vi "SetMCP.vi"(0 "Strings in":string[](array[string])=["C:\\CuspControl\\GPIB and Network\\Cusp\\MCPvolts.txt", "6723"], 1 "Dubs in":dbl[](array[numeric])=[0.0, 0.0, 0.0]) -> ()   [LabVIEW 2018]
panel:
  in  "Tab Control":enum32{"Variables", "Setup"}(tab)
  in  "Gain (Vout/Vcontrol)":dbl[](array[numeric])=[15.0, 208.0, 511.0]
  in  "mcpF, mcpB, phos (end)":dbl[](array[numeric])=[0.0, 0.0, 0.0] format="%0.2f"
  in  "mcpF, mcpB, phos (start)":dbl[](array[numeric])=[0.0, 0.0, 0.0] format="%0.2f"
  in  "upper limit":dbl[](array[numeric])=[100.0, 900.0, 3200.0]
  in  "lower limit":dbl[](array[numeric])=[-100.0, 0.0, 0.0]
  in  "MCPvolts":path=path "C:/CuspControl/GPIB and Network/Cusp/MCPvolts.txt"
  in  "ao lines":string[](array[string])=["ao5", "ao6", "ao7"]
  in  "subvi":bool=TRUE
  in  "gain file":path=path "C:/CuspControl/Cusp/Configuration/MCPgain.txt"
  # "DO NOT CHANGE GAIN"
  # "ao5\nao6\nao7"
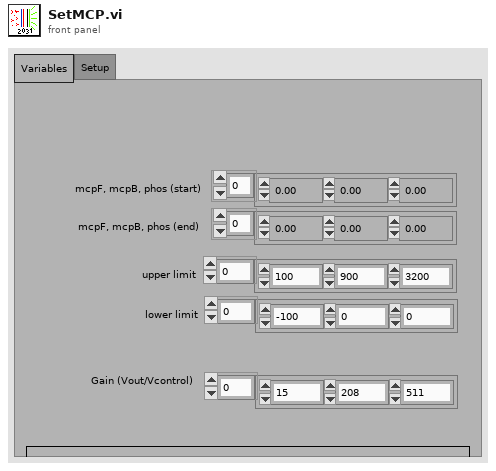
[diagram p1: front panel]
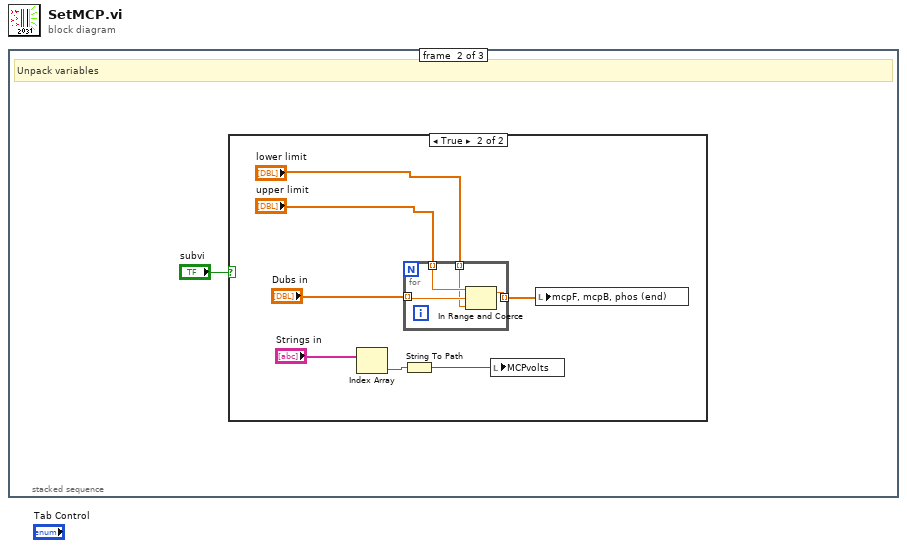
[diagram p0: block diagram]
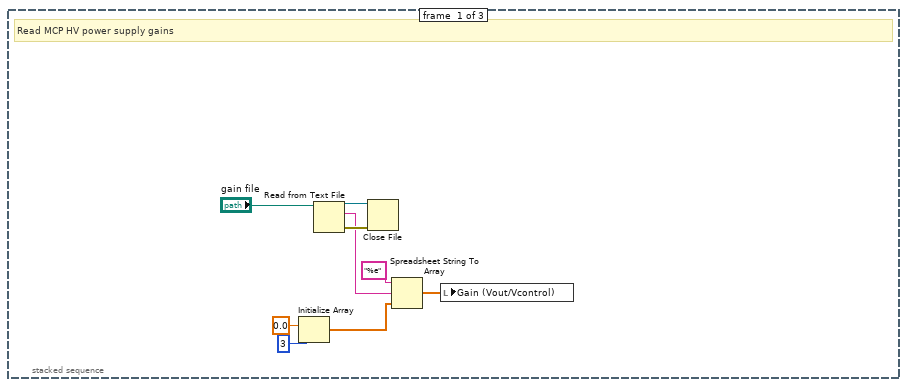
[diagram p2: hidden frame]
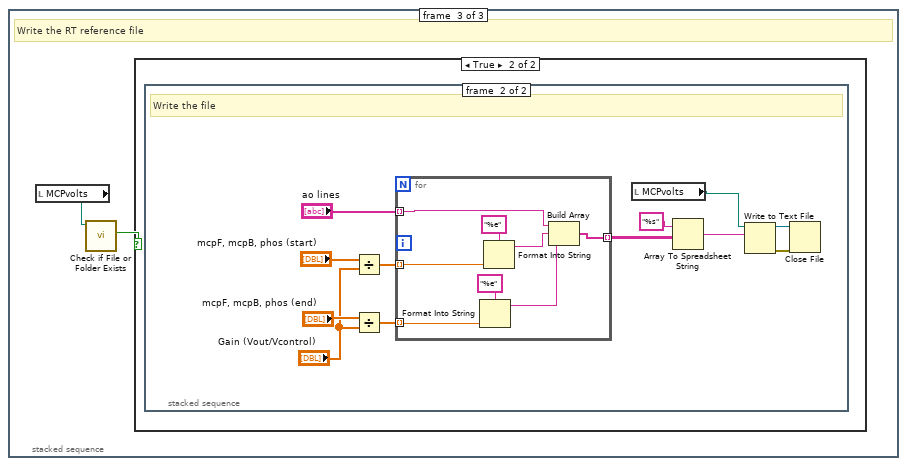
[diagram p4: hidden frame]
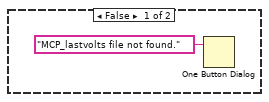
[diagram p5: hidden frame]
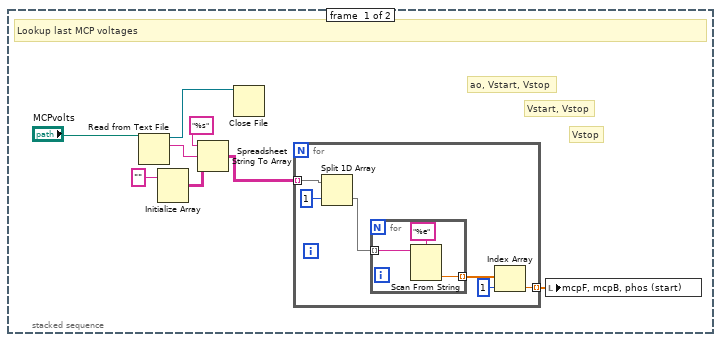
[diagram p6: hidden frame]
diagram:
  n1 = stacked-sequence {
    frame #0 {
      # "Read MCP HV power supply gains"
      n2 = Initialize Array(0.0 ("element"), 3 ("dimension size")) -> (w3:dbl[])
      n3 = Read from Text File(file (use dialog)="gain file") -> (refnum out=w8:refnum<file>, text=w6:string, error out=w7:errorcluster)  [unwired: 3 in, 1 out]
      n4 = Close File(refnum=w8, error in=w7) -> ()  [unwired: 2 out]
      n5 = Spreadsheet String To Array(format string="%e", spreadsheet string=w6, array type (2D Dbl)=w3) -> (array=w1:dbl[])  [unwired: 1 in]
      n6 = local write "Gain (Vout/Vcontrol)"(w1) -> ()
    }
    frame #1 {
      # "Unpack variables"
      n7 = case shown="True" "subvi" {
        frame False {
        }
        frame True {
          n8 = Index Array(array="Strings in") -> (element=w16:string)  [unwired: 1 in]
          n9 = for {
            tunnel: "Dubs in" -> [w21] mode=indexing
            tunnel: [w20] -> w13 mode=indexing
            tunnel: "upper limit" -> [w19] mode=indexing
            tunnel: "lower limit" -> [w18] mode=indexing
            n10 = In Range and Coerce(upper limit=w19, x=w21, lower limit=w18) -> (coerced(x)=w20:dbl)  [unwired: 1 out]
          }
          n11 = String To Path(string=w16) -> (path=w15:path)
          n12 = local write "MCPvolts"(w15) -> ()
          n13 = local write "mcpF, mcpB, phos (end)"(w13) -> ()
        }
      }
    }
    frame #2 {
      # "Write the RT reference file"
      n14 = local read "MCPvolts"() -> (w23:path)
      n15 = call <vilib>:"Check if File or Folder Exists.vi"("path"=w23) -> ("file or folder exists?"=w22:bool)  [unwired: 8 in, 2 out]
      n16 = case shown="True" w22 {
        frame False {
          n17 = One Button Dialog(message="MCP_lastvolts file not found.") -> ()  [unwired: 1 in, 1 out]
        }
        frame True {
          n18 = stacked-sequence {
            frame #0 {
              # "Vstop"
              # "Vstart, Vstop"
              # "ao, Vstart, Vstop"
              # "Lookup last MCP voltages"
              n19 = Read from Text File(file (use dialog)="MCPvolts") -> (refnum out=w27:refnum<file>, text=w28:string)  [unwired: 3 in, 2 out]
              n20 = Initialize Array("") -> (w30:string[][])  [unwired: 2 in]
              n21 = Spreadsheet String To Array(format string="%s", spreadsheet string=w28, array type (2D Dbl)=w30) -> (array=w32:string[][])  [unwired: 1 in]
              n22 = Close File(refnum=w27) -> ()  [unwired: 1 in, 2 out]
              n23 = for {
                tunnel: w32 -> [w38] mode=indexing
                tunnel: [w33] -> w26 mode=indexing
                n24 = Split 1D Array(array=w38, index=1) -> (second subarray=w36:string[])  [unwired: 1 out]
                n25 = for {
                  tunnel: w36 -> [w41] mode=indexing
                  tunnel: [w39] -> w35 mode=indexing
                  n26 = Scan From String(format string="%e", input string=w41) -> (output 1=w39:dbl)  [unwired: 3 in, 3 out]
                }
                n27 = Index Array(array=w35, index=1) -> (element=w33:dbl)
              }
              n28 = local write "mcpF, mcpB, phos (start)"(w26) -> ()
            }
            frame #1 {
              # "Write the file"
              n29 = Divide(x="mcpF, mcpB, phos (start)", y="Gain (Vout/Vcontrol)") -> (x/y=w45:dbl[])
              n30 = Divide(x="mcpF, mcpB, phos (end)", y="Gain (Vout/Vcontrol)") -> (x/y=w44:dbl[])
              n31 = for {
                tunnel: "ao lines" -> [w60] mode=indexing
                tunnel: w44 -> [w57] mode=indexing
                tunnel: [w59] -> w50 mode=indexing
                tunnel: w45 -> [w54] mode=indexing
                n32 = Format Into String(format string="%e", w57) -> (resulting string=w55:string)  [unwired: 2 in, 1 out]
                n33 = Format Into String(format string="%e", w54) -> (resulting string=w56:string)  [unwired: 2 in, 1 out]
                n34 = Build Array(w60, w56, w55) -> (w59:string[])
              }
              n35 = local read "MCPvolts"() -> (w42:path)
              n36 = Array To Spreadsheet String(array=w50, 3:"%s" ("format string")) -> (spreadsheet string=w47:string)  [unwired: 1 in]
              n37 = Write to Text File(file (use dialog)=w42, text=w47) -> (refnum out=w48:refnum<file>, error out=w49:errorcluster)  [unwired: 2 in, 1 out]
              n38 = Close File(refnum=w48, error in=w49) -> ()  [unwired: 2 out]
            }
          }
        }
      }
    }
  }
